vi "Nimbelink_Database_Get_Next_Address.vi"(0 "Work order":string, 5 "Error in (no error)":errorcluster) -> (14 "Duplicate serial numbers?":bool, 15 "Duplicate serial numbers":string[](array[string]), 19 "Error out":errorcluster)   [LabVIEW 2013]
panel:
  out "RecordSet 2":string[][](array[string])
  out "Distinct Passed Units Cnt":i32
  out "Passed Units Cnt":i32
  out "RecordSet":string[][](array[string])
  in  "ConnectionString":string="Provider=SQLOLEDB.1;Integrated Security=SSPI;Persist Security Info=False;Initial Catalog=Nimbelink;Data Source=DEVSERVER\\TESTDEPT"
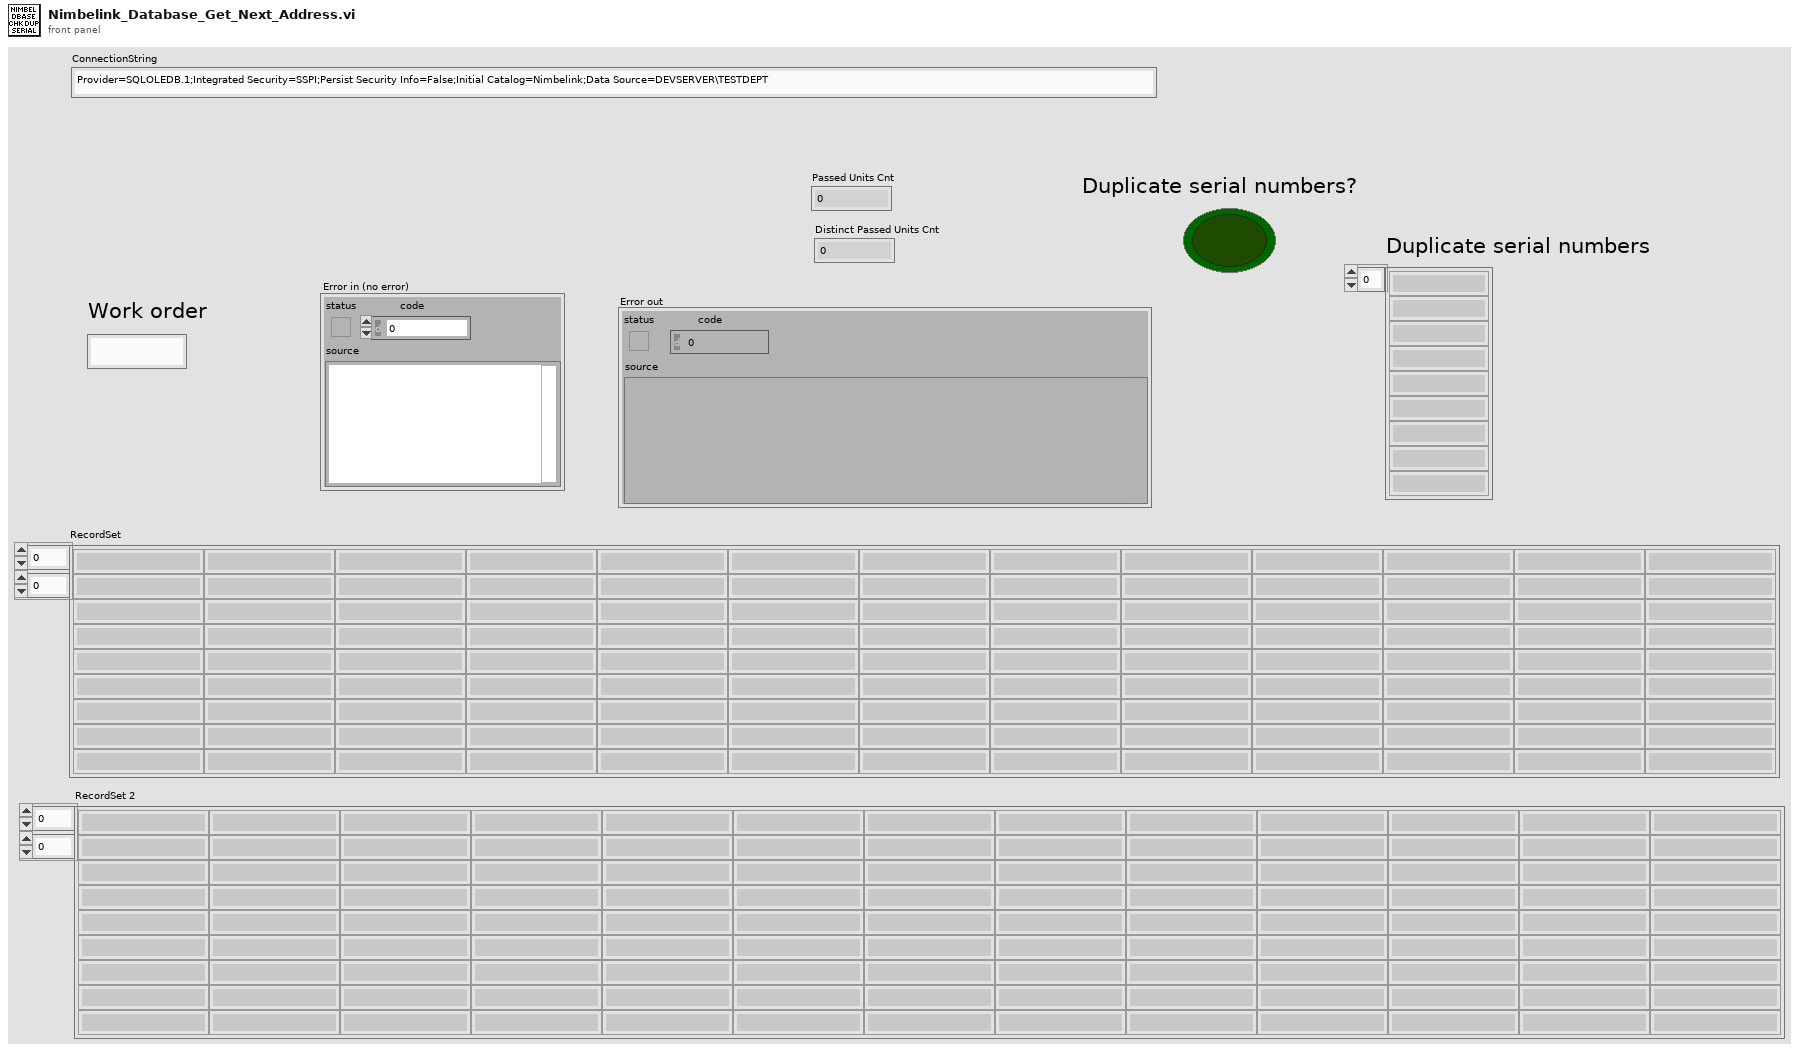
[diagram p1: front panel]
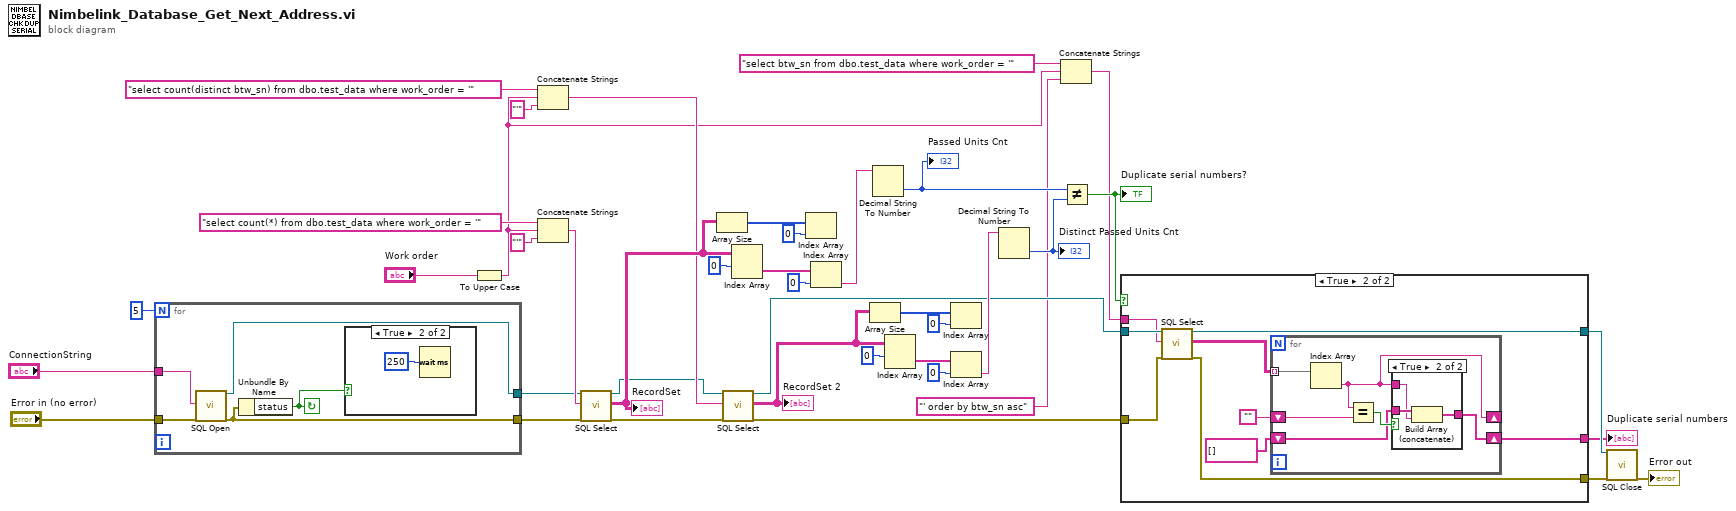
[diagram p0: block diagram]
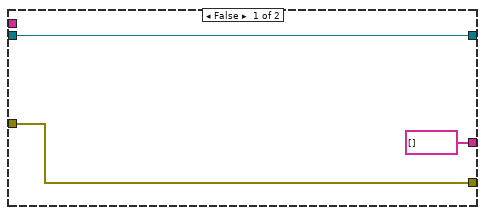
[diagram p2: hidden frame]
diagram:
  n1 = for {
    N: 5 -> [_]
    tunnel: "ConnectionString" -> [w46]
    tunnel: "Error in (no error)" -> [w45]
    tunnel: [w44] -> w27
    tunnel: [w43] -> w32
    stop <- w42 continue-if-true
    n2 = call "SQL Open.vi"("ConnectionString In"=w46, "Error in (no error)"=w45) -> ("Connection Out"=w44:refnum<k7>, "Error out"=w43:errorcluster)  [unwired: 16 in]
    n3 = Unbundle By Name(w43) -> ("status"=w42:bool)
    n4 = case shown="True" w42 {
      frame False {
      }
      frame True {
        n5 = Wait (ms)(milliseconds to wait=u32 250) -> ()  [unwired: 1 out]
      }
    }
  }
  n6 = To Upper Case(1:"Work order") -> (0:w4:string)
  n7 = Concatenate Strings("select count(distinct btw_sn) from dbo.test_data where work_order = '" ("string"), w4, "'" ("string")) -> (w17:string)
  n8 = Concatenate Strings("select count(*) from dbo.test_data where work_order = '" ("string"), w4, "'" ("string")) -> (w29:string)
  n9 = call "SQL Select.vi"("Connection In"=w27, "SQL Query"=w29, "Error in (no error)"=w32) -> ("Connection Out"=w15:refnum<k7>, "Data"=w33:string[][], "Error out"=w16:errorcluster)  [unwired: 14 in]
  "RecordSet" <- w33
  n10 = Array Size(array=w33) -> (size(s)=w34:i32[])
  n11 = call "SQL Select.vi"("Connection In"=w15, "SQL Query"=w17, "Error in (no error)"=w16) -> ("Connection Out"=w9:refnum<k7>, "Data"=w26:string[][], "Error out"=w8:errorcluster)  [unwired: 14 in]
  "RecordSet 2" <- w26
  n12 = Index Array(array=w33, index (row)=0) -> (element=w37:string[])  [unwired: 1 in]
  n13 = Index Array(array=w34, index=0) -> ()  [unwired: 1 out]
  n14 = Index Array(array=w37, index=0) -> (element=w39:string)
  n15 = Array Size(array=w26) -> (size(s)=w25:i32[])
  n16 = Decimal String To Number(string=w39) -> (number=w12:i32)  [unwired: 2 in, 1 out]
  "Passed Units Cnt" <- w12
  n17 = Index Array(array=w26, index (row)=0) -> (element=w22:string[])  [unwired: 1 in]
  n18 = Index Array(array=w25, index=0) -> ()  [unwired: 1 out]
  n19 = Index Array(array=w22, index=0) -> (element=w20:string)
  n20 = Decimal String To Number(string=w20) -> (number=w11:i32)  [unwired: 2 in, 1 out]
  "Distinct Passed Units Cnt" <- w11
  n21 = Concatenate Strings("select btw_sn from dbo.test_data where work_order = '" ("string"), w4, "' order by btw_sn asc" ("string")) -> (w2:string)
  n22 = Not Equal?(x=w12, y=w11) -> (x != y?=w10:bool)
  "Duplicate serial numbers?" <- w10
  n23 = case shown="True" w10 {
    tunnel: w9 -> [w49 w58]
    tunnel: w8 -> [w50 w59]
    tunnel: [w50 w51] -> w7
    tunnel: [w49 w52] -> w6
    tunnel: w2 -> [_ w57]
    tunnel: [string[] [] w53] -> w1
    frame False {
    }
    frame True {
      n24 = call "SQL Select.vi"("Connection In"=w58, "SQL Query"=w57, "Error in (no error)"=w59) -> ("Connection Out"=w52:refnum<k7>, "Data"=w56:string[][], "Error out"=w51:errorcluster)  [unwired: 14 in]
      n25 = for {
        tunnel: w56 -> [w65] mode=indexing
        shift-right: [w60] -> _
        shift-left: "" -> [w64]
        shift-right: [w61] -> w53
        shift-left: string[] [] -> [w62]
        n26 = Index Array(array=w65) -> (element=w60:string)  [unwired: 1 in]
        n27 = Equal?(x=w60, y=w64) -> (x = y?=w63:bool)
        n28 = case shown="True" w63 {
          tunnel: w62 -> [w66 w69]
          tunnel: w60 -> [_ w68]
          tunnel: [w66 w67] -> w61
          frame False {
          }
          frame True {
            n29 = Build Array (concatenate)(w69, w68) -> (w67:string[])
          }
        }
      }
    }
  }
  "Duplicate serial numbers" <- w1
  n30 = call "SQL Close.vi"("Connection In"=w6, "Error in (no error)"=w7) -> ("Error out"=→"Error out":errorcluster)  [unwired: 17 in]
